vi "Compute alpha(beta) Plot.vi"(8 "Error In":errorcluster, 10 "Phasor Parameters":T1={"Display Parameters"={"# Points"=0, "Ramp Type"=enum."Linear", "Type of Series"=enum."1-Exp Decays", "Min tau"=0.0, "Max tau"=0.0, "Include 0"=FALSE, "Include Infinity"=FALSE}, "Phasor Parameters"={"Harmonic Frequency"=0.0, "Use f* = 1/D Frequency"=FALSE, "Calibrated Phasor"=FALSE, "Calibration Lifetime"=1e-09, "Phasor Calculation"=enum."Direct Sum", "SEPL Type"=enum."UC", "# Gates"=1.0, "Square Gate Width"=1e-09, "Show Ticks"=FALSE}, "Decay & IRF Parameters"={"Lifetime"=0.0, "IRF Offset"=0.0, "IRF Period"=0.0, "Normalized Decays"=FALSE, "IRF Model"=enum."Dirac", "IRF Parameter 1"=0.0}, "Gate Parameters"={"First Gate Start"=0.0, "Use Gate Center"=FALSE, "Gate Width"=0.0, "Gate Step"=0.0, "# Gates"=0.0, "Gate Type"=enum."Square", "Edge Width"=0.0, "Top Slope"=0.0, "Reversed Sawtooth?"=FALSE, "Analytical Computation"=FALSE, "Integration"=enum."Item 0", "Tolerance"=1.0, "# Steps"=1.0, "Type of User-defined Function"=enum."Gate", "Use Gate Step"=FALSE}, "Detector Parameters"={"Frames/Image"=0, "Gates/Frame"=0, "Bits/Frame"=0, "Multiplicity"=0, "Incident Signal"=0.0, "Poisson Signal"=FALSE}} {"Detector Parameters"."Frames/Image" min=1; "Detector Parameters"."Multiplicity" min=0; "Detector Parameters"."Bits/Frame" min=1; "Detector Parameters"."Gates/Frame" min=1; "Gate Parameters"."# Steps" min=0.0; "Gate Parameters"."Tolerance" min=0.0; "Gate Parameters"."Top Slope" min=0.0; "Gate Parameters"."Edge Width" min=0.0; "Gate Parameters"."Gate Step" min=0.0; "Gate Parameters"."# Gates" min=0.0 step=1.0; "Gate Parameters"."Gate Width" min=0.0; "Decay & IRF Parameters"."Lifetime" min=0.0; "Decay & IRF Parameters"."IRF Period" min=0.0; "Phasor Parameters"."Square Gate Width" min=0.0; "Phasor Parameters"."# Gates" min=0.0; "Phasor Parameters"."Calibration Lifetime" min=0.0; "Phasor Parameters"."Harmonic Frequency" min=0.0; "Display Parameters"."Min tau" min=0.0; "Display Parameters"."Max tau" min=0.0; "Display Parameters"."# Points" min=1 step=1}, 11 "alpha(beta) Graph Refnum":refnum<vi>) -> (0 "Error Out":errorcluster, 2 "Max Lifetime":dbl[unit], 3 "Min Lifetime":dbl[unit])   [LabVIEW 2019]
uses:
  SEPL Parameters.ctl
  Phasor Explorer Display Parameters.ctl
  Type of Series.ctl
  Phasor Explorer Phasor Parameters.ctl
  Phasor Calculation Type.ctl
  SEPL Type.ctl
  Phasor Explorer Decay Parameters.ctl
  IRF Model.ctl
  Phasor Explorer Gate Parameters.ctl
  Gate Type.ctl
  Type of User-defined Function.ctl
  Phasor Explorer Detector Parameters.ctl
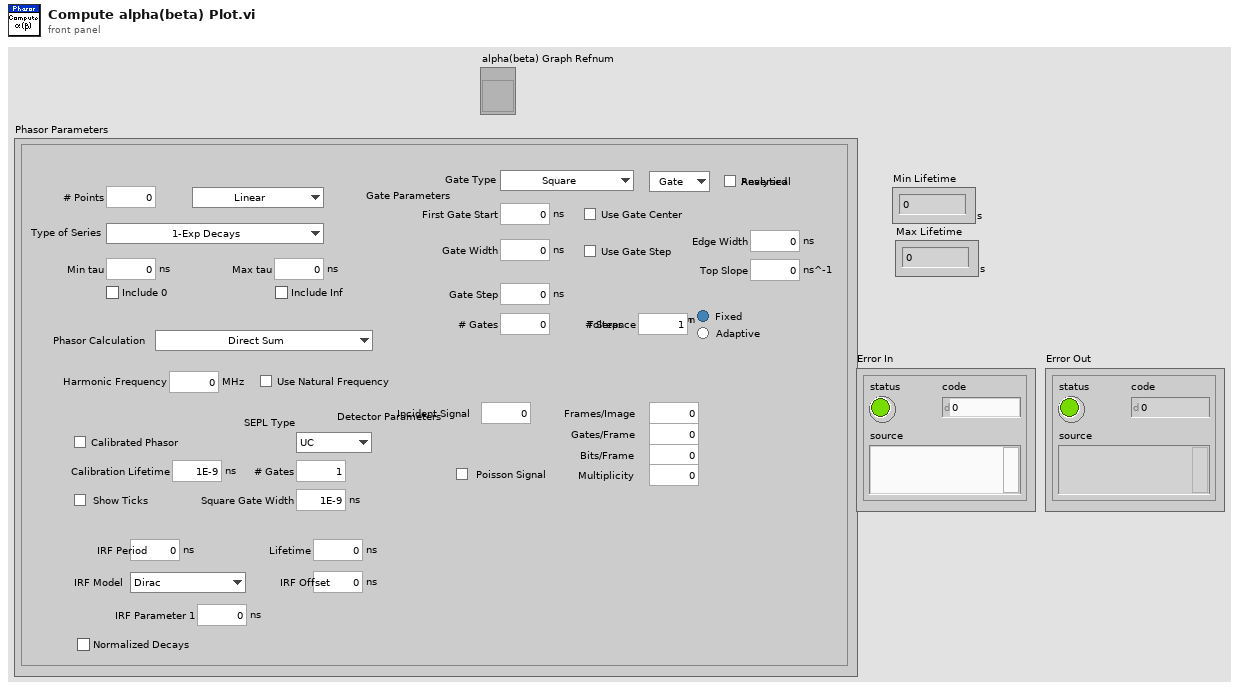
[diagram p1: front panel]
types:
  T1 = typedef "SEPL Parameters.ctl" = cluster{"Display Parameters":T2, "Phasor Parameters":T4, "Decay & IRF Parameters":T7, "Gate Parameters":T9, "Detector Parameters":T12}
  T2 = typedef "Phasor Explorer Display Parameters.ctl" = cluster{"# Points":i32, "Ramp Type":enum16{"Linear", "Logarithmic"}, "Type of Series":T3, "Min tau":dbl[unit], "Max tau":dbl[unit], "Include 0":bool, "Include Infinity":bool}
  T3 = typedef "Type of Series.ctl" = enum16{"1-Exp Decays", "Linear Combination of 1-Exp"}
  T4 = typedef "Phasor Explorer Phasor Parameters.ctl" = cluster{"Harmonic Frequency":dbl[unit], "Use f* = 1/D Frequency":bool, "Calibrated Phasor":bool, "Calibration Lifetime":dbl[unit], "Phasor Calculation":T5, "SEPL Type":T6, "# Gates":dbl, "Square Gate Width":dbl[unit], "Show Ticks":bool}
  T5 = typedef "Phasor Calculation Type.ctl" = enum16{"Direct Sum", "Analytical Formula"}
  T6 = typedef "SEPL Type.ctl" = enum16{"UC", "L_N", "L_N[W]", "L_X"}
  T7 = typedef "Phasor Explorer Decay Parameters.ctl" = cluster{"Lifetime":dbl[unit], "IRF Offset":dbl[unit], "IRF Period":dbl[unit], "Normalized Decays":bool, "IRF Model":T8, "IRF Parameter 1":dbl[unit]}
  T8 = typedef "IRF Model.ctl" = enum16{"Dirac", "Exponential"}
  T9 = typedef "Phasor Explorer Gate Parameters.ctl" = cluster{"First Gate Start":dbl[unit], "Use Gate Center":bool, "Gate Width":dbl[unit], "Gate Step":dbl[unit], "# Gates":dbl, "Gate Type":T10, "Edge Width":dbl[unit], "Top Slope":dbl[unit], "Reversed Sawtooth?":bool, "Analytical Computation":bool, "Integration":enum32{"Item 0", "Item 1"}, "Tolerance":dbl, "# Steps":dbl, "Type of User-defined Function":T11, "Use Gate Step":bool}
  T10 = typedef "Gate Type.ctl" = enum16{"Square", "Finite Edge Square", "Finite Edge, Tilted Top Square", "Triangle", "Sawtooth", "User-defined"}
  T11 = typedef "Type of User-defined Function.ctl" = enum16{"Gate", "IRF"}
  T12 = typedef "Phasor Explorer Detector Parameters.ctl" = cluster{"Frames/Image":i32, "Gates/Frame":i32, "Bits/Frame":i32, "Multiplicity":i32, "Incident Signal":dbl, "Poisson Signal":bool}
  T13 = typedef "Gate Definitions.ctl" = cluster{"First Gate: t1":ext, "Gate Width: W":ext, "Gate Step: d":ext, "# Gates: G":ext, "Use Gate Center":bool, "Frames/Image: F":i32, "Gates/Frame: L":i32, "Bits/Frame: q":i32, "Multiplicity: p":i32, "Gate Type":T10, "Gate Edge s":ext, "Gate Top Slope":ext, "Reversed Sawtooth?":bool, "Computation":bool, "User-defined Gate":T14, "Tolerance":ext, "Integration":enum32{"Item 0", "Item 1"}, "# Steps":ext, "Type of User-defined Function":enum32{"Gate", "IRF"}}
  T14 = typedef "XY Plot Data.ctl" = cluster{"X Array":dbl[], "Y Array":dbl[]}
  T15 = typedef "Decay Definiton.ctl" = cluster{"offset: t0":ext, "period: T":ext, "lifetime: tau":ext, "Incident Signal: I":ext, "Normalized Decays":bool, "IRF Model":T8, "IRF Parameter 1":ext, "Poisson Signal":bool}
  T16 = typedef "Phasor (g, s).ctl" = cluster{"g":dbl, "s":dbl}
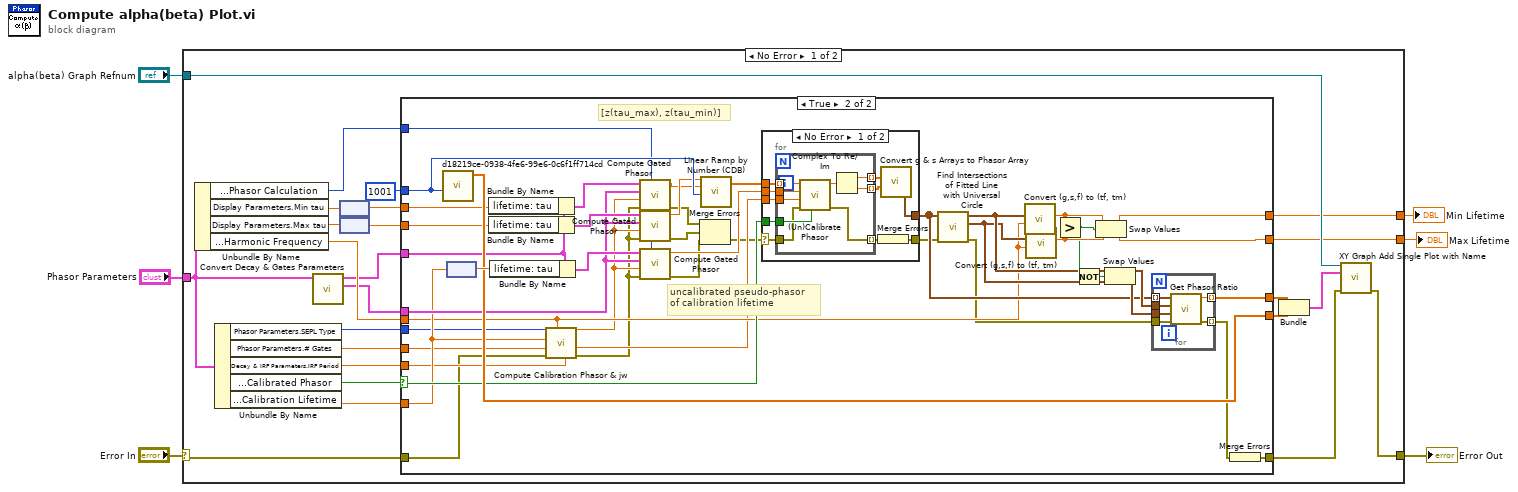
[diagram p0: block diagram]
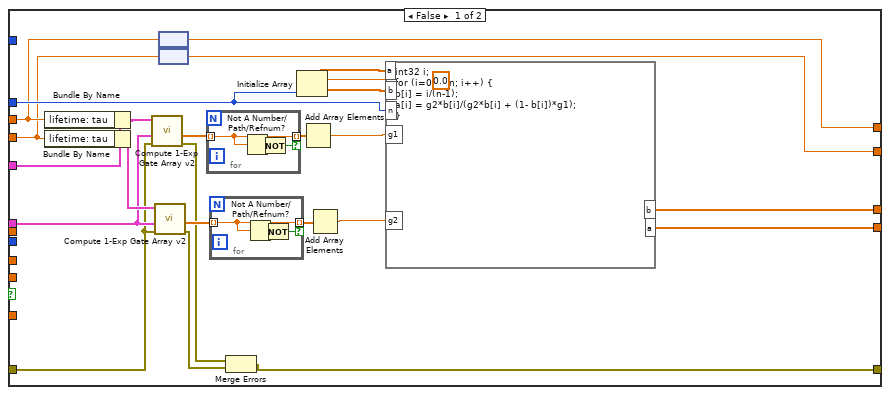
[diagram p2: hidden frame]
diagram:
  n1 = case shown="No Error" "Error In" {
    selector: "Error In" -> [w8 w131]
    tunnel: "Phasor Parameters" -> [w15 _]
    tunnel: "alpha(beta) Graph Refnum" -> [w28 _]
    tunnel: [w27 w131] -> w3
    tunnel: [w19 _] -> w2
    tunnel: [w18 _] -> w1
    frame No Error {
      n2 = Unbundle By Name(w15) -> ("Phasor Parameters.Phasor Calculation"=w12:T5, "Display Parameters.Min tau"=w29:dbl[unit], "Display Parameters.Max tau"=w30:dbl[unit], "Phasor Parameters.Harmonic Frequency"=w20:dbl[unit])
      n3 = Unbundle By Name(w15) -> ("Phasor Parameters.SEPL Type"=w11:T6, "Phasor Parameters.# Gates"=w10:dbl, "Decay & IRF Parameters.IRF Period"=w9:dbl[unit], "Phasor Parameters.Calibrated Phasor"=w14:bool, "Phasor Parameters.Calibration Lifetime"=w13:dbl[unit])
      n4 = call "Convert Decay & Gates Parameters.vi"("Phasor Parameters"=w15) -> ("Gates Definitions"=w16:T13, "Decay Definition"=w17:T15)  [unwired: 9 in]
      n5 = node(w29) -> (w25:dbl)
      n6 = node(w30) -> (w24:dbl)
      n7 = case shown="True" w14 {
        selector: w14 -> [_ w81]
        tunnel: w17 -> [w52 w89]
        tunnel: w25 -> [w42 w90]
        tunnel: w24 -> [w40 w88]
        tunnel: w16 -> [w50 w85]
        tunnel: [w45 w92] -> w23
        tunnel: [w44 w91] -> w22
        tunnel: 1001 ("dimension size") -> [w43 w84]
        tunnel: w20 -> [_ w75]
        tunnel: [w41 w100] -> w19
        tunnel: [w39 w99] -> w18
        tunnel: w13 -> [_ w76]
        tunnel: w12 -> [_ w77]
        tunnel: w11 -> [_ w73]
        tunnel: w10 -> [_ w72]
        tunnel: w9 -> [_ w62]
        tunnel: w8 -> [w34 w60]
        tunnel: [w32 w65] -> w7
        frame False {
          n8 = Bundle By Name(cluster=w52, "lifetime: tau"=w42) -> (w51:T15)
          n9 = Bundle By Name(cluster=w52, "lifetime: tau"=w40) -> (w53:T15)
          n10 = call "Compute 1-Exp Gate Array v2.vi"("Error In"=w34, "Gates Definitions"=w50, "Decay Definition"=w51) -> ("Error Out"=w31:errorcluster, "Gate Image Array"=w38:ext[])  [unwired: 4 in, 3 out]
          n11 = call "Compute 1-Exp Gate Array v2.vi"("Error In"=w34, "Gates Definitions"=w50, "Decay Definition"=w53) -> ("Error Out"=w33:errorcluster, "Gate Image Array"=w36:ext[])  [unwired: 4 in, 3 out]
          n12 = node(w42) -> (w41:dbl[unit])
          n13 = node(w40) -> (w39:dbl[unit])
          n14 = for {
            tunnel: w38 -> [w59] mode=indexing
            tunnel: [w59] -> w37 mode=indexing if=w57
            n15 = Not A Number/Path/Refnum?(number/path/refnum=w59) -> (NaN/Path/Refnum?=w58:bool)
            n16 = Not(x=w58) -> (.not. x?=w57:bool)
          }
          n17 = for {
            tunnel: w36 -> [w56] mode=indexing
            tunnel: [w56] -> w35 mode=indexing if=w54
            n18 = Not A Number/Path/Refnum?(number/path/refnum=w56) -> (NaN/Path/Refnum?=w55:bool)
            n19 = Not(x=w55) -> (.not. x?=w54:bool)
          }
          n20 = Merge Errors(w31, w33) -> (w32:errorcluster)
          n21 = Initialize Array(0.0 ("element"), w43) -> (w46:dbl[])
          n22 = Add Array Elements(numeric array=w37) -> (sum=w49:ext)
          n23 = Add Array Elements(numeric array=w35) -> (sum=w48:ext)
          n24 = formula code="int32 i;\nfor (i=0; i<n; i++) {\nb[i] = i/(n-1);\na[i] = g2*b[i]/(g2*b[i] + (1- b[i])*g1);\n}"("g1"=w49, "g2"=w48, "b"=w46, "a"=w46, "n"=w43) -> ("b"=w45:dbl[], "a"=w44:dbl[])
        }
        frame True {
          # "[z(tau_max), z(tau_min)]"
          # "uncalibrated pseudo-phasor\nof calibration lifetime"
          n25 = call "d18219ce-0938-4fe6-99e6-0c6f1ff714cd.vi"("# Steps (1)"=w84) -> ("Ramp"=w91:dbl[])  [unwired: 8 in, 2 out]
          n26 = node(w76) -> (w103:dbl)
          n27 = Bundle By Name(cluster=w89, "lifetime: tau"=w90) -> (w87:T15)
          n28 = Bundle By Name(cluster=w89, "lifetime: tau"=w88) -> (w86:T15)
          n29 = Bundle By Name(cluster=w89, "lifetime: tau"=w103) -> (w104:T15)
          n30 = call "Compute Calibration Phasor & jw.vi"("Laser Period"=w62, "Harmonic frequency"=w75, "Error In"=w60, "# Gates"=w72, "Calibration Lifetime"=w76, "Calibration Phasor Type"=w73) -> ("Error Out"=w61:errorcluster, "z (tau_cal)"=w71:cdb, "i 2 pi f (GHz)"=w74:cdb)  [unwired: 3 in]
          n31 = call "Compute Gated Phasor.vi"("Phasor Calculation Type"=w77, "Error In"=w61, "j 2 pi f"=w74, "Gates Definitions"=w85, "Decay Definition"=w87) -> ("Error Out"=w70:errorcluster, "phasor"=w79:cxt)  [unwired: 4 in, 1 out]
          n32 = call "Compute Gated Phasor.vi"("Phasor Calculation Type"=w77, "Error In"=w61, "j 2 pi f"=w74, "Gates Definitions"=w85, "Decay Definition"=w86) -> ("Error Out"=w69:errorcluster, "phasor"=w80:cxt)  [unwired: 4 in, 1 out]
          n33 = call "Compute Gated Phasor.vi"("Phasor Calculation Type"=w77, "Error In"=w61, "j 2 pi f"=w74, "Gates Definitions"=w85, "Decay Definition"=w104) -> ("Error Out"=w68:errorcluster, "phasor"=w82:cxt)  [unwired: 4 in, 1 out]
          n34 = Merge Errors(w70, w69, w68) -> (w64:errorcluster)
          n35 = call "Linear Ramp by Number (CDB).vi"("# Steps"=w84, "End"=w79, "Start"=w80) -> ("Ramp"=w83:cdb[])  [unwired: 7 in, 1 out]
          n36 = case shown="No Error" w64 {
            selector: w64 -> [w107 w124]
            tunnel: [w114 _] -> w93
            tunnel: w83 -> [w113 _]
            tunnel: w82 -> [w112 _]
            tunnel: w81 -> [w109 _]
            tunnel: w71 -> [w108 _]
            tunnel: [w105 w124] -> w63
            frame No Error {
              n37 = for {
                tunnel: w113 -> [w122] mode=indexing
                tunnel: w112 -> [w121]
                tunnel: w108 -> [w120]
                tunnel: [w119] -> w111 mode=indexing
                tunnel: [w118] -> w110 mode=indexing
                tunnel: w109 -> [w117]
                tunnel: w107 -> [w116]
                tunnel: [w115] -> w106 mode=indexing
                n38 = call "(Un)Calibrate Phasor.vi"("Calibrated Phasor"=w117, "Error In"=w116, "Target Phasor"=w120, "Calibration Phasor"=w121, "Phasor in"=w122) -> ("Error Out"=w115:errorcluster, "Phasor out"=w123:cxt)  [unwired: 5 in]
                n39 = Complex To Re/Im(x + iy=w123) -> (x=w119:ext, y=w118:ext)
              }
              n40 = Merge Errors(w106) -> (w105:errorcluster)
              n41 = call "Convert g & s Arrays to Phasor Array.vi"("s"=w110, "g"=w111) -> ("Phasor Array"=w114:T16[])  [unwired: 8 in]
            }
            frame Error {
            }
          }
          n42 = call "Find Intersections of Fitted Line with Universal Circle.vi"("Error In"=w63, "Phasor Array"=w93) -> ("Error Out"=w67:errorcluster, "Intersection 2"=w96:cluster{"x":dbl, "y":dbl}, "Intersection 1"=w97:cluster{"x":dbl, "y":dbl})  [unwired: 5 in, 2 out]
          n43 = call "Convert (g,s,f) to (tf, tm).vi"("Phasor Harmonic Frequency"=w75, "Phasor (g, s)"=w97) -> ("Phase Lifetime"=w102:dbl[unit])  [unwired: 8 in, 1 out]
          n44 = call "Convert (g,s,f) to (tf, tm).vi"("Phasor Harmonic Frequency"=w75, "Phasor (g, s)"=w96) -> ("Phase Lifetime"=w101:dbl[unit])  [unwired: 8 in, 1 out]
          n45 = Greater?(x=w102, y=w101) -> (0:w98:bool)
          n46 = Not(x=w98) -> (.not. x?=w78:bool)
          n47 = Swap Values(12:w102, 13:w98, 14:w101) -> (1:w100:dbl[unit], 3:w99:dbl[unit])
          n48 = Swap Values(12:w97, 13:w78, 14:w96) -> (1:w95:cluster{"x":dbl, "y":dbl}, 3:w94:cluster{"x":dbl, "y":dbl})
          n49 = for {
            tunnel: w95 -> [w130]
            tunnel: w94 -> [w129]
            tunnel: w93 -> [w128] mode=indexing
            tunnel: [w127] -> w92 mode=indexing
            tunnel: w67 -> [w126]
            tunnel: [w125] -> w66 mode=indexing
            n50 = call "Get Phasor Ratio.vi"("Error In"=w126, "Reference Phasor 2"=w129, "Reference Phasor 1"=w130, "Phasor"=w128) -> ("Error Out"=w125:errorcluster, "Phasor Ratio"=w127:sgl)  [unwired: 6 in]
          }
          n51 = Merge Errors(w66) -> (w65:errorcluster)
        }
      }
      n52 = Bundle("b"=w23, "Ramp"=w22) -> (w26:cluster{"b":dbl[], "Ramp":dbl[]})  [unwired: 1 in]
      n53 = call "XY Graph Add Single Plot with Name.vi"("XYGraph Ref in"=w28, "Plot"=w26, "error in (no error)"=w7) -> ("error out"=w27:errorcluster)  [unwired: 9 in, 3 out]
    }
    frame Error {
    }
  }
  "Error Out" <- w3
  "Min Lifetime" <- w2
  "Max Lifetime" <- w1
